vi "Fetch Multi Eval Meas List PERR Peak Results.vi"(7 "Window Position (Low)":i32(ring) items=["Low", "High"], 8 "error in (no error)":errorcluster, 9 "Result Type (Current)":i32(ring) items=["Current", "Average", "Extreme", "Standard Deviation"], 10 "Instance (1)":T1=1, 11 "VISA resource name":refnum<visa-resource-name>) -> (0 "error out":errorcluster, 1 "PERR Peak Results":dbl[](array[numeric]) format="%^.3e", 2 "Reliability":i32, 3 "VISA resource name out":refnum<visa-resource-name>)   [LabVIEW 2015, in "Rohde&Schwarz CMXP NR FR2 Measurement.lvlib"]
doc: "Returns phase error peak values for low and high EVM window position, for all measured list mode segments.\n\nAttributes:\nRSCMXPNRFR2M_ATTR_FETCH_MULTI_EVAL_MEASUREMENT_LIST_PERR_PEAK_HIGH_AVERAGE_RESULTS\nRSCMXPNRFR2M_ATTR_FETCH_MULTI_EVAL_MEASUREMENT_LIST_PERR_PEAK_HIGH_CURRENT_RESULTS\nRSCMXPNRFR2M_ATTR_FETCH_MULTI_EVAL_MEASUREMENT_LIST_PERR_PEAK_HIGH_EXTREME_RESULTS\nRSCMXPNRFR2M_ATTR_FETCH_MULTI_EVAL_MEASUREMENT_LIST_PERR_PEAK_HIGH_STANDARD_DEVIATION_RESULTS\nRSCMXPNRFR2M_ATTR_FETCH_MULTI_EVAL_MEASUREMENT_LIST_PERR_PEAK_LOW_AVERAGE_RESULTS\nRSCMXPNRFR2M_ATTR_FETCH_MULTI_EVAL_MEASUREMENT_LIST_PERR_PEAK_LOW_CURRENT_RESULTS\nRSCMXPNRFR2M_ATTR_FETCH_MULTI_EVAL_MEASUREMENT_LIST_PERR_PEAK_LOW_EXTREME_RESULTS\nRSCMXPNRFR2M_ATTR_FETCH_MULTI_EVAL_MEASUREMENT_LIST_PERR_PEAK_LOW_STANDARD_DEVIATION_RESULTS\n\nRemote-control commands:\nFETCh:NRMMw:MEAS<i>:MEValuation:LIST:MODulation:PERRor:PEAK:HIGH:AVERage?\nFETCh:NRMMw:MEAS<i>:MEValuation:LIST:MODulation:PERRor:PEAK:HIGH:CURRent?\nFETCh:NRMMw:MEAS<i>:MEValuation:LIST:MODulation:PERRor:PEAK:HIGH:EXTReme?\nFETCh:NRMMw:MEAS<i>:MEValuation:LIST:MODulation:PERRor:PEAK:HIGH:SDEViation?\nFETCh:NRMMw:MEAS<i>:MEValuation:LIST:MODulation:PERRor:PEAK:LOW:AVERage?\nFETCh:NRMMw:MEAS<i>:MEValuation:LIST:MODulation:PERRor:PEAK:LOW:CURRent?\nFETCh:NRMMw:MEAS<i>:MEValuation:LIST:MODulation:PERRor:PEAK:LOW:EXTReme?\nFETCh:NRMMw:MEAS<i>:MEValuation:LIST:MODulation:PERRor:PEAK:LOW:SDEViation?"
uses:
  <instrlib>/Rohde&Schwarz CMXP NR FR2 Measurement/Rohde&Schwarz CMXP NR FR2 Measurement.lvlib
  <instrlib>/Rohde&Schwarz CMXP NR FR2 Measurement/Private/_Instance.ctl
  <instrlib>/Rohde&Schwarz CMXP NR FR2 Measurement/Private/rsidr_core.llb/rsidr_core.lvlib
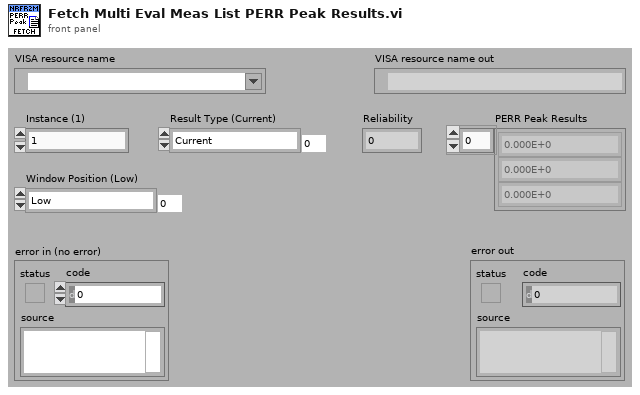
[diagram p1: front panel]
types:
  T1 = typedef "Rohde&Schwarz CMXP NR FR2 Measurement.lvlib/_Instance.ctl" = i32
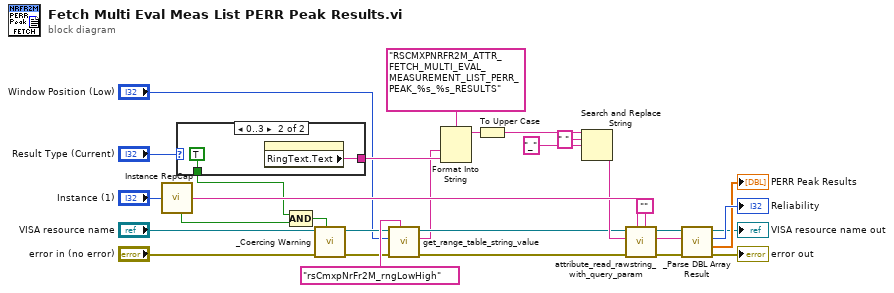
[diagram p0: block diagram]
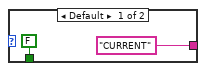
[diagram p2: hidden frame]
diagram:
  n1 = call <instrlib>:"Instance RepCap.vi"("Instance In"="Instance (1)") -> ("In Range?"=w26:bool, "RepCap Identifier Out"=w29:string)  [unwired: 1 in]
  n2 = case shown="0..3" "Result Type (Current)" {
    tunnel: ["CURRENT" w33] -> w27
    tunnel: [FALSE TRUE] -> w3
    frame Default {
    }
    frame 0..3 {
      n3 = property on="Result Type (Current)" class="Ring (strict)"() -> ("RingText.Text"=w33:string)  [unwired: 2 in, 2 out]
    }
  }
  n4 = Compound Arithmetic op=AND(w3, w26) -> (w25:bool)
  n5 = call <instrlib>:"_Coercing Warning.vi"("In Range?"=w25, "error in (no error)"="error in (no error)", "VISA resource name"="VISA resource name") -> ("error out"=w7:errorcluster, "VISA resource name out"=w8:refnum<visa-resource-name>)  [unwired: 7 in]
  n6 = call <instrlib>:"get_range_table_string_value.vi"("Range Table ID in"="rsCmxpNrFr2M_rngLowHigh", "error in"=w7, "I32 input"="Window Position (Low)", "VISA resource name"=w8) -> ("error out"=w5:errorcluster, "String Value out"=w1:string, "VISA resource name out"=w4:refnum<visa-resource-name>)  [unwired: 5 in]
  n7 = Format Into String(format string="RSCMXPNRFR2M_ATTR_FETCH_MULTI_EVAL_MEASUREMENT_LIST_PERR_PEAK_%s_%s_RESULTS", w1, w27) -> (resulting string=w28:string)  [unwired: 2 in, 1 out]
  n8 = To Upper Case(1:w28) -> (0:w23:string)
  n9 = Search and Replace String(input string=w23, search string=" ", replace string="_" ("replace string (\"\")")) -> (result string=w20:string)  [unwired: 5 in, 3 out]
  n10 = call <instrlib>:"attribute_read_rawstring_with_query_param.vi"("Query Parameter (None)"="" ("Empty String Constant"), "Repeated Capability"=w29, "error in"=w5, "Attribute ID"=w20, "VISA resource name"=w4) -> ("error out"=w19:errorcluster, "Raw String out"=w18:string, "VISA resource name out"=w17:refnum<visa-resource-name>)  [unwired: 4 in]
  n11 = call <instrlib>:"_Parse DBL Array Result.vi"("error in (no error)"=w19, "Input String"=w18, "VISA resource name"=w17) -> ("error out"=→"error out":errorcluster, "Results"=→"PERR Peak Results":dbl[], "Reliability"=→"Reliability":i32, "VISA resource name out"=→"VISA resource name out":refnum<visa-resource-name>)  [unwired: 5 in]
